vi "18_2.vi"() -> ()   [LabVIEW 2018]
panel:
  out "spreadsheet string":string="8\t*\t(\t3\t+\t6\t)\t*\t8\t*\t(\t2\t+\t4\t)\r\n"
  out "Value Out":u64=3456
  out "Operators 2":string[](array[string])=["8", "*", "(", "3", "+", "6", ")", "*", "8", "*", "(", "2", "+", "4", ")"]
  out "Array":u64[](array[numeric])=[86918496042, 35, 42033600, 5155488000, 1435, 231660, 320460800, 186, 2584012800, 1224608, 20280, 96, 28684, 4634, 288, 8798976, 155520, 2051315, 32682, 473128, 6966, 5107502736, 53084160, 1260, 204918052, 6900, 37044, 4092, 14580, 513010, 90, 123, 24752, 7920, 27216, 1360800, 28, 40960, 19296, 2934392832000, 33, 67469025, 9465, 114520, 5100, 637119, 654, 30, 2095120, 213355479168, 11827211, 6909, 26, 11328, 911680, 12644, 33, 207176, 4759, 1114344, 29, 12496275, 1118880, 520, 146480, 23520, 985600, 170311680, 156909312, 18, 180, 8456616, 50544, 75888, 6450672000, 1714006008, 12600, 36310, 24, 6604431, 982652496, 41920, 23328, 8400, 24524800, 32580, 1425, 2843, 27876736, 576, 114057, 17892, 18, 144720, 5882, 177600, 500, 4368, 190728, 303156, 39618, 75, 8640, 18, 1497233808, 112, 1188, 657720, 176904, 15750720, 3680, 832944, 1020096, 14696640, 29428, 918600, 23328, 4095, 125244, 19684, 7700400, 349930800, 2484, 3060, 9014208, 53844, 32480, 1190, 16224024, 5552064, 23997024, 176, 10032336, 41606712, 48, 159667200, 759974400, 318780, 2204, 87611717952, 608107500, 125, 126, 2880, 38, 8064, 30305, 500957184, 14675814, 19989504, 2278, 3030660, 212284816, 4105092, 536, 52995735016224, 7632, 18467906688, 9367068, 570381, 3933, 44335104, 546, 15120, 91887348, 34699, 2421, 252, 62008139, 240, 68094, 516, 123480, 81518400, 84, 85, 32702292, 560, 189, 115200, 83175, 49, 6480, 8603364, 3732, 282640, 48, 204880, 3594384, 340, 314230, 4608, 1890, 102920, 255143, 83520, 50, 124800, 47382618729600, 38, 311216400, 9856, 152611279793280, 3740, 24, 58432, 22804, 1168, 1200558240, 243000, 3123394014, 155, 1049280, 11383672, 18360, 4050, 1306384, 16698, 1392, 29664, 1400, 42912, 12096, 218601, 20352, 11520, 208, 290306, 10080, 51417, 32, 10320, 302702400, 35426, 380160, 1650, 1616630404200, 1725456, 6048, 12980, 34819572, 13600651680, 3616, 58, 21735, 294, 144, 59346, 590733000, 1636752, 138240, 56026441240, 1643, 1028160, 1430, 36000, 88185240, 530838400, 18304, 6921193, 5250, 8, 2002910, 240, 21345009840, 928, 12355200, 606060, 189800, 109188, 1312, 3512008281600, 6977998264320, 44528, 2898, 82560, 1271808, 55399939, 270, 139689930240, 918778, 31299840, 178560, 343245, 137511, 270, 62974800, 109192050, 9036, 5040, 15271200, 449592, 116701568, 38088, 1260, 269954916, 2388, 46824960, 6028, 173892, 12348, 24570, 20790, 814, 1834, 4651101, 272268, 799029, 58480, 68510, 3149120, 3224592, 303408, 368640, 29694467, 2690552148480, 30249, 1068480, 54966739968, 137280, 2640, 1071616, 70025904, 232190, 1470, 790, 2352, 3636, 4368, 53032320, 60984, 52564909320, 30151, 1751137542, 13272600, 10969, 48934553310720, 160524000, 4352, 31, 2450, 453648, 468, 257, 6426, 21560, 3466935, 648, 6552, 2536, 93148, 6538860, 41472000, 17988, 1366740, 816, 718502400, 228750, 13547520, 33564, 48681, 78624, 98385477120, 1826496, 26880, 321672, 23294304, 2205, 248371200, 8709606, 16496865, 276, 1451526, 18630, 14871, 152460, 14136304, 420, 945, 5265, 3456]
  out "sum":u64=320536571743074
  in  "Input":string="(7 * (7 * 6 * 4 + 3)) * 3 + ((8 + 5 * 3 + 7 + 8) + 3 * (2 + 9 * 5 + 7 * 5 * 6) * 2 + 3 * 9) + (4 + 5 + 5 * 2 + 2) + ((5 + 6 + 9 + 6) + 3 + 4 * 6 * 5)\n7 * 5\n(9 * (9 + 7) * 7 + (4 + 5 * 5 + 2 + 3) + 3) * 7 * 5 + 8 + (4 + (7 + 9 + 6 * 9) * 2)\n((6 + 4) * 6 * (5 + 3) * 9 * (3 * 5 * 5 * 9 * 4 + 9) * 4) * 2 * 8 + 9\n7 * 7 + (9 + 2 * 9 + 9)\n9 + (7 * 7 * 5 * 9 * 7) * 2 + 3 * 3\n5 * (5 * (8 * 4) * 7 + 8 + 7) * (5 * (4 * 3 * 5 + 2 * 5) + (6 * 6 * 7 * 2 + 2) + 4) + (5 + 4 * 7 + 5 * 9 + 9) * 2\n((7 + 3 + 8) + (2 + 6 * 4 * 5)) + 8\n8 * (6 * 7 + 3 * (8 * 5 * 2 * 4)) * (3 + (5 + 5 + 6) * (4 * 3 + 7 * 5 + 7) + (3 * 5 * 9 * 3)) + 8\n6 + 4 + 8 + 4 * ((3 + 5 * 8) + 7 * 7 * 8 * 7 * 2)\n3 * (9 + 4) * (9 + 2 + 6 + 5) + 4 * (7 * 2) + 6\n4 * 6 + (8 + 3) + 7\n2 + (8 * (5 + 6 * 5) + 9 * 7 + (7 * 7)) + 5 + 5\n(8 + (5 * 7 * 3 + 6) + 8) * 8 + 6\n8 * 6 * 6\n8 * 6 + (9 + 4 * 5 * 3) * 9 * (4 * 2 + 6 + 7 + 4 * 8)\n(5 * 9 * 8 * 9 * 6) * 8\n7 * 5 + ((2 * 7 * 5 + 2 + 6 + 3) * 9) * 5 + ((2 * 2 * 4 + 3) * 5)\n(2 + 3 * 4 * (2 + 4 * 9 + 8) * 8) + 6 + 8 + 7 * 2\n3 + 7 + (3 * 4 * (8 * 6 + 8 * 8 * 2 + 9)) * 4\n9 * 9 + 9 + (3 * 7 * 9 * 4)\n(7 * 7 + (2 * 5 * 8) * 4) * 9 + (9 + 4 * 8 * (9 + 3 * 5 * 4 * 7 * 4)) + 3 * 3\n7 + 6 + 3 * 8 * 4 * (9 * 4 * (5 + 7 * 2 * 8 + 7 * 8))\n(7 + 2) * 5 * 8 + 6 * 2\n9 + 4 + (5 + (7 * 7 * 9 + 5) + 6 * 5 + 2 * (4 * 7 * 7 + 8 * 5 * 5)) * 2 + 2\n8 + 2 * 2 * (2 + (2 + 7 + 7 * 7 * 3) + 7)\n3 + 4 * (3 + 3 * 3 + 4) * 9 * 6 + 8\n((4 + 4 + 6) + (5 * 5 + 4 * 9 * 5) + 5) + 2 * 2\n9 * 5 * 6 * 2 + 6 + (2 * 9 + (2 * 3 + 4))\n(3 * 9) + 2 * (2 * 5 + 7 + 9 * 7 * 6) + 5 * 5 * 2\n7 + 3 + 5 * 6\n7 + 5 + (2 * 8 + (6 * 6) + 6) + (4 + 7)\n2 * (9 + 5 * 3 + 5 + 5 + 4) * (3 + 4 + 3 + 5 + 2 + 7) + 2 * 2\n(4 * 5 + 6 * 3 + (5 * 3)) * 5 + 5\n9 + 8 + 7 * (7 + 9 + 2 * 2 + 7) * 7\n3 * 3 * ((4 + 3 * 4 * 2 * 2 * 6) * (9 + 6) * 3) * 5\n9 + 6 + 7 + 6\n8 * (4 * 8 * 8 * 7 + 4 + 9)\n2 + (7 * 9 * 2) + 6 * 6 * 4 * 6\n((4 * 6 + 7 + 9 * 4) + 9) * 4 * ((6 * 3 + 3 + 9 * 7) * 8 * 4 * 5 * (2 * 6 * 8 * 5 + 5 * 3)) * 7\n(4 * 7) + 5\n6 + 9 * 6 + 9 + ((5 + 7 * 5 * 8) + 7 + 7 + 8 * (2 + 8 * 2 * 4 * 7 + 9) * 7)\n6 + 3 + (9 + 6 * (4 + 7 + 4 * 6 * 7)) + 6\n5 * 7 * (4 * 6 * (3 + 8 + 6 * 8)) + 8\n(5 * 6) * 8 + 2 * 3 + (7 + 4 + 3)\n3 + 4 * 9 * 2 + (7 + (5 * 9 * 7 + 7 * 4) * 4) + 3\n2 * 9 + ((3 + 5 + 2 + 9 * 9 + 6) + 4 + (6 * 4) + 2) + 3\n3 + 6 + (3 + 6 + 8 + 2 + 2)\n8 * ((8 * 6) + (7 + 2 * 2 * 2 + 4 * 3) * (9 + 8 + 4 * 8) + 8 * 4) + 2\n9 + 4 * (7 * (2 * 4 + 9 * 3 + 7) * 8 + (4 * 3 * 9 + 9 * 5 + 7) + 9 * (6 * 4 * 2)) + ((5 + 6 + 7 * 9 * 6 + 6) + (6 * 2 + 8 + 9 + 4 + 4) + (8 * 5 * 2 + 6 + 7) * 5 + 3) * 9 * 8\n9 + 2 + (5 + 3 * 2 * (7 + 4 * 5 * 5 + 3 * 7) * 8 * (5 * 6))\n7 * (3 + 3 + 7 * 7 * 9) + (2 + 5 * 6 * 4)\n9 + 8 + 9\n8 * (7 + (5 * 7) + (7 + 3) * 2 + 7) + 4 * 3\n2 * (2 * 6 + 5 * 7) * 2 + (3 + 3) * ((2 * 3 + 2) + (5 * 3 * 4 + 8 * 2))\n4 * (3 + 7 + 6 + 8 + 3 + 6) + 8 + (2 * 3 * (5 * 2 + 6 + 5 * 8))\n2 + 5 + 3 + 2 + 4 + (2 + (6 + 4) + 5)\n2 * (4 * 4) + (5 + 2 * (4 + 2 * 2 + 4) * 4 + (5 * 9 * 9) + 2)\n(6 + 9 + (3 + 5 * 3) + 4 * 2 * 2) + 7 + ((6 * 6 + 4 * 5 * 5 + 4) + 5) + ((8 + 4 + 9 * 8 * 9 + 2) + (7 + 2 + 9) + 4) + 5\n7 * 3 + (6 + (8 * 5) * 6 * 8) * 2 * 9 * 4\n9 + 9 + 9 + 2\n(7 * 9 * 2 + 8 * 7 * 4) + 9 + (9 * 6 * 9 + 7) * 3 * (9 * 5 * 5)\n4 * 7 * ((7 + 9 * 5 * 4 + 7 * 4) + (2 + 3 + 5 * 4 + 2) + (2 + 5 * 8 * 5 * 5 + 6)) * 6\n5 + 8 * (9 + (9 + 3 + 9 + 5 + 5))\n(3 * 7 * 2 * 3 + (8 + 8 + 3 * 9)) + 8 + 8 * 6 + 8 + 6\n9 + 4 + 8 * (7 * 8 + 8 + 4 * 8)\n2 * 9 + 2 * (5 + 3) * 2 * (5 * 5 * 8 + (3 + 4 + 4 + 5) + 4 * 4)\n5 * 7 + 2 * ((2 * 8 * 8 + 8 * 2 * 7) * 6 * 7 + 7 + 2) * 2 + 9\n4 * (6 * (6 * 3 * 3)) * (7 * 5 * 4 * 2 * (5 + 5 + 8 * 3)) + 7 + 7 * 8\n3 * 2 + 4\n9 + 6 * 2 * 4 + 2\n((5 * 5 + 3 + 7 * 2) * 2 * 5 + (9 + 9)) + 3 + 6 * (9 + 8) * 8 * 9\n4 * (8 + 2 + 3 * 9 * 6) * 6 * 3\n2 * (9 * 6 + (8 + 6 * 4) * (5 * 5) + 9 * 2)\n6 + (3 * (6 * 6 + 4 + 5) + 3 * 5 * 4 + (6 + 9 + 4 * 5 * 3)) + 6 * (3 + (6 + 5 + 5 + 6) * 8 + 8 * 4) * 4 + 6\n9 * 9 * 2 + (6 * 4 * 2 + 4 * 7 * 9) * 7 + ((5 + 6 + 7 + 7) * (7 * 3 + 9) + 9)\n(2 + (6 + 8 + 6 * 5 + 5) + 8 * 5) * 9 + 3\n2 * 9 + 2 + (9 * (4 + 6 + 4 + 2) * 9 * 5 + 7 + 2)\n8 + 6 + 4 + 6\n3 + ((6 * 4 + 2 + 4 + 3 + 8) * (4 * 3) * (9 + 4 * 6 + 2 * 7 * 6)) + 5 + 7\n3 * (8 * 4 + 9 + 4) * 7 * 2 + ((5 + 9 * 6 * 4 * 4) * 8 * 4 * (6 + 2))\n((8 * 7 + 6) * 3 + 2 + 5) + 8 * 5 * 8\n(3 * 2 * 6 * 3 * 2) * 6 * 2 * 9\n(4 * 8 * 3 + 5) + (8 + 9) + 7 * 7 + 3 * 3\n(2 + 7 * (7 * 8)) + 8 + (6 * (4 * 8) * 4 * 2 * 8) * 4 * ((7 + 8 + 4 + 3 + 6) * 4 + 9 + 4) + 3\n((7 + 2 + 3 * 3) * 5 * 5 + 4) + 9 * 2 + 7 + 9 + 2\n(6 + (2 + 7)) * 4 + 7 + 8 * 5\n(9 * 8) + (8 + (2 + 4 + 5 + 6 * 9) + 2 * (8 + 9))\n2 * (9 + 8) * 8 * ((7 * 6 + 7 * 3) + 2 + 5 * (7 * 2 + 7 + 8) + 3 * 3) + 8\n4 * 6 + 6 + 4 * 9\n(2 + 4 + 5 + 3 + 6) + 3 * 3 * 3 + (5 * 2 * 9 + 6 * 6 + 5)\n7 * 5 + (6 + 2 * 2 * 8 + 5) * 6 + 6\n(5 + 8 + 2) + 3\n3 + 3 * 5 * ((3 + 8 + 5 + 9) * 4 + 4 * 4 + 4) + 8 * 3\n2 + (5 + 5 + (6 * 5 * 2 * 8) * 4 + 8)\n8 + (5 * 7 * 2 * 2) * (7 + 9 * 5) * 2 + 9 + 4\n((9 * 9) + 6 + 4 + 9) * 5\n5 + 3 * ((4 + 8) + 9 * 2 * 6 + 7)\n6 + 7 + 5 * (2 + 9 * 4 * 5 * 7 + 5) + 9 * 4\n(7 * 2 + 4 + (8 * 8 + 2 * 5 * 3 * 6)) + (4 + 4 * 3 + 7) + 4 * 6\n2 * (5 * 9 * (5 + 3 * 5) * 5 + 6) + 4 + 5\n5 * (4 + 7 + 4)\n9 * 7 + 8 + 4 + (6 * (6 * 2 * 4 + 9)) + 5\n6 * 3\n(5 * 6 + 2 * (2 + 5 * 6 * 4 + 9 + 2)) + (4 + 3 * (9 * 9 + 4 * 8 * 8 * 9) * 4) * (8 + 7 + (4 + 8 * 2 + 4) * 9)\n8 * 5 + 9\n7 + 4 * 9 * 6 + 6\n9 + 6 * (8 * (7 * 6 + 2 + 4 + 6 + 9) * 2 + 2 + 2 + (7 + 7 + 9))\n6 * (7 * 6 * 6) * 9 * 6 + 7\n(5 * 7 + 9) * 7 + ((4 * 5 + 3) * 5 * (3 + 8 * 7) + 2 + 3 * (7 + 6 + 2)) + (3 * 5 * 5) + 2\n4 * 2 * 2 * 2 * (6 + 4 + 9 + 4 * 5)\n((9 * 7 + 7) + 8 * 7) * 4 + (7 + 9 * 9) * 6\n8 * (6 * (8 + 4) + (5 + 6) * 6) * 7 + 4 * 7 * 2\n(7 + 7 * (8 * 5 + 4)) * 5 * (3 * 6 * 2 * 3 * 9) * 3\n4 + (7 * 5 * 3 * 5 + 3 * 5) * 7\n(6 + 5 + 6 * 3 * (6 * 4 + 6)) + 2 * 5 * 9 + 3 * 5\n3 * (6 + 3 + 5 * 3) + 6 * 3 + (7 + 8) * 9\n(3 + 8 + (5 * 4 + 4 + 7) + 5 * 2) + 2 + 5 + 6 * 9 + (4 + 2 + 6)\n9 * 8 + (3 + (4 + 2 * 8 + 7 * 5 + 3) + (3 * 3) * 3 + (2 * 8))\n7 * 4 + (3 + 7 + 6 + 4 * (3 * 6) * 2) + ((5 + 5 * 5) + 6 + 2 * (2 * 3 * 3 + 3))\n9 * 5 * (6 + (2 * 3)) + (3 * 4 + 3 + 9 + 6) + (9 + 5 + 2 + (3 * 4 * 9 * 9 * 5) + 2 * 7) * 5\n(6 + 9 * 4 + 5 * 4 * (8 + 2 * 4 * 2 * 3)) + 4 * 9 + 6 * (4 * 5 * 9)\n9 * 7 + (2 + (6 + 3) + (4 * 3 + 9) + 9) + 8 + 9 * 3\n3 * (8 + 7 + 7 + 8) * (5 + 5 + 2 + 6 + 9 + 7)\n7 + (7 * 5 + 3 * 4 * 9 + 2) * (8 * 6 + (5 + 2) + 6) * 4 + (6 * 3) + 2\n(4 * 5 + 7 + 3 * (7 * 8) + 8) + 6 * 2 + 9 + 3\n7 * 4 * 8 * (7 + 5 + 2) + (8 * 8 * 2) + 3\n7 + 7 * (6 + (4 * 7 + 3 + 2 + 7) + 3)\n2 + (8 + (5 + 9 + 2 * 6 * 6 + 8) * 8 + 2 * (5 * 2 + 8) * 4) + 2 * 6\n(4 * 9 * (7 * 6 * 9 + 8 * 6) * 9) * 2 * 2\n3 + (8 + 2 + (2 + 3 * 2) * 6 + (5 * 8 * 8 * 8 + 2 + 3)) * 4 * (9 + 3) * 6\n8 + 3 * (3 + 5) + 3 + 5\n4 + ((9 * 5 * 2 + 7 + 5) + 6 + 3 + 6 * (7 * 6) + 6) * 2 * 3 * (3 * 9 + 9)\n((4 * 9) * 8 * 6) + 8 * 8 + 6 + ((6 + 4 + 7) * (2 + 2 * 4 * 9) + 3 + (5 * 9 + 9 * 9 + 5) + 2)\n(8 * 4) + (8 + 8)\n((4 + 5 + 2 * 4 * 7 + 3) * 6 * (4 * 6 + 8) * 9 * (9 + 7 + 5 + 3)) * 5\n8 * 2 + 8 + (7 * (8 + 2 + 6 * 7 + 9) + (5 + 9 + 3) + 6 * 6) * (8 + (4 * 2 + 4 + 7 * 5) + 2 * 6) * 5\n(2 * 5 + (8 * 7 + 9 + 2 + 2)) * 2 + (8 * (2 + 4) + 4 * 5 + 7) + 4\n4 + (2 + (4 * 3 * 9) * 5 * 4)\n((3 + 4) * 7 + 6 + (5 * 3 * 8 + 8 * 9) * 3 + 6) + 8 * 4 * ((7 + 4 * 3) * (6 + 9 + 9 * 4 * 7) + 9 + 5 + 2 + (5 + 8 * 4 * 6 + 4 * 8))\n4 * (9 * 5 * (5 * 7 * 7 + 4)) * 5 * (5 * 7 + (4 * 5) * 4 + 9)\n5 + (8 * 6 + 8) + 8\n7 + (8 + 6) * 4 + 2\n(3 * (9 + 6 * 8)) * 8\n3 + 6 + 4 + ((5 + 4 * 2) + 7)\n7 * 3 + 5 * (2 * 5 + 4) * 8\n5 * 5 + (6 * (8 + 5) * 7) * 7 + 4\n7 + 9 + (2 + (3 + 8 + 4) + 9 * 2 + 6) * (7 + (3 + 6 * 8 + 8 * 7) + 9 * 3 * 8 + (9 * 6 + 2 + 8 + 4 * 4))\n6 * (2 * 8 + 3 + 5 + 5) + (3 + (8 * 2 * 3) * (2 + 9 * 8 * 5 + 3) + 4 + 7) * 7 + (5 * 5 + 7)\n(2 * 2 * 6 * 4 * 9 + (9 * 5 + 7 * 4 + 6 * 2)) * 4 + (4 + (8 * 2 + 3 + 6))\n2 + (8 + 4 * 8 + 3) * 6 + 7 + 4\n(6 + 6 * (2 * 5 * 5 * 4 * 5 * 4) + 8 * 7 * 3) + 5 + (3 * 6 + 3 * 7) + 5 + 5 * 3\n2 * (8 + 2 + 6 * (9 * 9 * 9 + 4 * 2 * 7) * 3 * (4 + 6 * 3 + 8 + 4)) + 8\n(6 * 7 + 8 * 6 * 7 + (5 + 9 * 3 + 6 + 9 * 5)) + 2 * 6\n(7 + 2 * 4 + 3) + 4 * 5 + 3\n((7 * 7 + 2 + 7) + (3 + 3 + 5 + 9 * 3 + 2) * (2 * 4 * 7 + 6 * 3)) * (2 + (7 + 4 + 3 * 9 + 4 * 5) * 4 + 3 * (5 + 8 * 3)) + 5 + (2 + 8 * 2 * 8 * (6 * 7 + 4 + 5)) * (3 * (7 * 6 * 3 * 8)) + 7\n3 * 4 * ((8 + 8 + 9) * 6 + 6 + 7 + 6) + 8 + 3\n(6 + (7 * 4) + (9 + 6 + 3 * 9)) + 2 * (4 + 6 * 5 + (2 + 8) * 5 + 9) + 3 * (6 + 8 + 8 * (7 * 8 * 3 * 2 + 2 + 8))\n(9 + 8 * 4 + (5 * 8 + 7 * 2 * 8 * 9) * 8 + 9) * 3\n9 + ((5 * 3 + 6) + (8 + 6 * 6 + 7 + 2 + 8) * 8 + 5 + (9 + 8 + 2 * 9 + 2)) * 7\n((8 + 2 + 6 + 3) * 8 + 5 + 8 + 2) * 9\n(6 + (4 * 4 * 7 * 2 + 6) * 4 + 2 * 8 * (6 + 2 * 8)) * 2 * 8\n3 * (4 + 3 + 3 + (3 * 7 * 7)) + 6 + 7 + 4 + 8\n(6 * 8 + 7) * 8 * 9 + 8 + 4\n(7 * 7) * 2 + (8 * 7) + 4 * (5 * 2 * (3 + 4 + 7 * 8 * 3) * 9) + 6\n7 + (9 * (6 + 8 * 7 + 6 * 3) + 4) * 4 + 3\n6 + 3 * ((2 + 2 + 3 + 9 + 9 + 8) * 6 + 2) + 5\n3 * 6 * 6 + 2 + 2 + (2 * 2)\n6 + (4 + 9 * (5 + 9 * 4 * 6 + 6) + 4 * 6 * (2 * 7 * 7 * 4 + 8)) + 5\n((2 + 6) + 2 + 5) + 7 + 3 + 5 * 3 + 5\n(6 * (2 + 8 + 7) + 4 * (2 + 8) * 9) + 9 * 6\n(2 * (9 * 4 * 3 * 2) + (4 + 4 * 3 + 2)) + 4\n(6 + 4 * (5 + 9)) + 7 * 7 * 8 * 5 * 3\n(3 + (5 + 4 * 3 + 9)) * 2 * (9 + 6 * 6 * (7 + 8 + 2 * 5) * 8 * 6)\n8 + 6 * 6\n8 + (8 * 9) + 5\n8 + (7 * (6 + 8) * 7 * (5 * 7 * 8 * 7) + (8 + 4 + 6 * 9 + 8) + 4) + (6 * 4) * 3 * 7\n9 + 4 + 3 * 7 * 5\n(8 + 9) + 6 + 4 * 7\n5 * (4 * 6 + 4 + 2 * (5 * 2 * 2 * 8)) * 3\n3 * 3 + 2 + ((8 + 5 + 4 + 8 + 8) * 7 * 6 + 9 * 8)\n9 + (8 + (8 + 9) + 7 + 8)\n(8 + 2) + (2 + 5 + 7) + 6 * 6 * 6 * 6\n5 + 7 + (5 + 4 * (5 * 6 + 3 + 3) + (7 * 9 * 5 * 6 * 6 + 3) * 8) * 7\n6 + ((7 * 3) * 6 * 5 + 5 + (3 + 3 + 9)) + (6 * 2 + 6 + 9 + (2 + 4 * 3 * 4) + 7)\n8 * 5 + (9 * 2 * 7 * 2 * 6 + 8) * 2 + 2 + 6\n6 * 8\n(2 * 3 + 5 + (8 + 6 * 8 * 7 * 2)) * 3 + 2 + 6 + 2 * 5\n(7 + 6 * (2 + 2 * 4 * 9 + 7 * 5) * 4 + 2) + 4 * (9 + 6) + (9 + 5) + 7\n5 * (3 + 7 + 7 * 4)\n2 * ((2 * 7 * 8 * 4 * 3 + 7) + 6 + 3) * 5 * 7\n8 * 4 + 7 + (6 * 4 + 3 + 2) + 7 * 8\n7 * 9 + (2 * 9 * 2) * 6\n8 + (6 * (2 + 8) + 9) + (7 + 6 + 6 * (8 * 3 * 5 * 5 * 9) + 3 + 7) + 8\n2 + 5 * 4 + (4 * (3 + 7 * 5 + 8) * 8 + 2) + 3 * 7\n(8 * (9 * 7 + 9 + 9 + 4) * 3 + 2) * 8\n4 + (6 + (2 + 4 * 6) + 4)\n(8 * (4 + 6 + 2 * 6 + 7)) * 9 + 8 + 3 * 5\n((2 * 7 + 3 * 5) * (5 + 7 + 7 + 3 * 7 * 3) * 8) * 2 * ((2 * 9 * 4 * 6 + 4) + 6 + (8 * 5 * 4 * 5 * 6 * 8) + 7 * (9 * 6 + 7 * 3 + 4 + 7)) + 9\n6 + 8 + (3 * 3 + 2) + 5 + 4\n5 * 6 + 6 * 5 * ((3 + 5 * 8 + 4 * 8) * 9 * 9 + 6 * 4 + 6) + (4 * 7 * 5 + 9 + 7)\n2 * 7 * (4 * 7 + (4 + 7 + 4 + 3 * 2 + 7) + 7)\n((8 + 3 * 6 * 6 + 4) + (9 + 5 + 3 * 3) + 7 * (3 * 4 + 4 + 9 * 4 + 6) + (8 + 5 + 2 * 2 * 5)) * 8 * 6 * 7 + ((5 + 6 + 2 * 4 + 2) * (9 + 8 + 9) + 6 + (6 * 5 * 9 + 7) * 4 * 6) * 7\n4 * 5 * (9 * 3) + (9 + 6 + 5 * 8)\n3 * 8\n9 + 2 * (7 + (2 + 9) * 9) + 4 * 4 * 8\n(8 + 4 + 7 * 2 + 8 * (8 + 7 * 4 + 4)) + 4\n4 + 8 + ((7 * 9 + 9) + 3 + 2 + 3) * 8\n(6 + (4 + 3 + 8 + 6 * 8)) * (5 + 9 * (5 + 2 * 7 + 8) + (6 * 7 * 4 + 2 * 5) + 4 * 9) * 8 * 5\n8 + 3 + 4 * 9 * ((4 * 9 + 3 + 6) + 3 * 3 + 9) * 2\n6 + ((3 * 2) * (4 + 9 + 9 * 5 * 2) * (2 * 8 + 4 * 7 + 4 + 8)) * 5 + (9 * 4 * 6 + 6 * 4 + 8)\n2 + (5 + 4 * 8) + (9 * 9)\n8 * 3 + 7 * 3 + ((2 * 2 + 6 * 3) * 3 * 7 * 8 + 5) + 9\n4 * 7 + ((6 + 7 * 3 * 4 + 8) * 2 + 6 + (4 * 6 + 9 + 6 * 8 * 3) + 3 * 3) + 3\n5 * (9 * 9 + (7 + 6 + 2 + 9 + 9 + 9)) * 8\n5 + 4 * 2 + 7 * (5 * 5 + 2 + 3)\n2 * 2 + 6 + ((2 + 2 + 5) * 6 * (2 + 7 + 3 * 9) * 5 + 9 * 8)\n((2 * 4 + 7) + 9 * 8) + 5 * 6 * 2 + 9\n6 + ((7 * 9 * 9 + 2) * 2)\n6 * (7 + (4 + 7 * 2) * 5 + 2 + 7) + 6 * 7 + 5\n8 * (6 * 8 + (7 + 2 + 7) + 3) + 7 + 6\n(7 * 2 * 3 * 7) + 4 * 3 + 6 * 9 + 7\n8 * 7 * (8 * 9 * 3)\n9 + (9 * 4 * (9 + 3 * 5 + 9 + 9) * 8 + 5 + 9)\n6 * (9 * 2 * 9 + 6 + 9 + 8) + (6 * 9 * 5) + 2 * 4\n2 * 5 * (7 + 8 + 3 + 8 + 6 * 4) * 4 + 5\n2 * 2 * (4 + 3) + 2 + 4 * 4\n(6 * (9 * 6 + 2 * 2) * 4 * 3 * 4 * 7) + 2\n(2 * 5) * 3 + 3 * 3 * 7 * 8\n3 + 6 + ((6 * 6) * (9 + 8 * 2) * 7 + 5 + 9 * 2)\n9 + 7 + (2 * 8)\n(8 * 7) + (8 + 6 * 7 + (3 * 9 + 6) * 6 + 8) + (4 * 2 * 9)\n2 + 2 + 2 + 9 * ((4 + 5 * 7 * 5 * 4 * 7) * (9 + 9) + 4 * 4 + 9) * 8\n4 + 2 + ((6 + 8 * 4 + 7) * 7 + 3 * 9 + (9 + 5))\n7 + 8 * (3 * (3 + 9 + 6 * 5) + 6 * 8) * 7 + 4\n8 + 7 * (2 * (5 * 7)) + (4 * 3 + 7)\n(2 + 8 * 7) + ((8 * 9 * 3 + 3 + 5 * 7) * 2 * (9 + 6 * 3 * 5) * 4 * (4 + 6 * 6 + 4 * 9) * 3) * 6 + 4 * 4 + 2\n3 * (9 + 4 + (9 + 5 + 8 + 6 * 3 * 4) * 8 + (9 * 3 + 8 + 4 + 7)) * 8\n(4 + 4 * (4 * 7)) * 2 + 7 * 3\n((4 * 9) * (9 + 6 + 9 * 8 + 7)) + 6 + 7 + 7\n6 + ((9 * 5 + 9 + 6 * 6 + 4) * 7 + (9 + 5 + 5) * 9 + 3) * (5 * 9) + 8 + 9\n(3 + 8 * (7 * 3 * 4)) * (6 * (6 + 4) + (9 + 8) * (2 * 5 + 4) + (8 + 5 * 6 + 5 * 2 + 2)) * 6 + 9 + (7 + 6 * 5) + (5 + 4 + (6 + 8 * 2) * 2)\n4 * ((6 * 8 + 7 * 6 + 4) + 4)\n((5 * 6) + 4) + (9 + 4 + 9) + 2\n5 * 9 * 7 * 6 + (9 * 7)\n5 + (2 + 7) * 5 + 9 + 7\n6 * 2 * 8 + 4\n(3 + 2 * 4 + 8) + ((7 * 5 + 7 * 2 * 8) + 7 + 2) * 6 * 2 + 5\n(2 * 5) * (3 * 9 * 4 * 8 + 5 * 3) * ((9 + 5 * 6 * 3) + 3 * 7 + 4) * 5\n((3 + 6 * 3) * (4 + 9 * 5 * 6 + 4 * 7)) + ((8 * 7 * 2 + 7) + 5 * 6) * 6 + 7\n(8 + 4 * 8 * 8) * 9 * 9 + 7 + 4\n(7 * 9 + 5) * 5 + (9 + 4 + 4 + (7 * 9 * 2 * 8 * 2 + 9)) * ((7 * 5 * 7 * 3 * 7) * 5 * 2) + 8\n5 + (6 * (8 + 9) * 7 + 9) + 3 + 3\n8 + 8 * (6 * 5 * (3 + 5 + 9 * 2 * 9 * 7))\n5 * (4 + 7) * 5 + 7 + 8 + 6\n3 * ((5 + 6 + 2 + 7) * 4 * 6) * 5 * 5\n(6 + 3 * (9 * 9 * 7 * 8 * 9 + 9) + 5) * 8 * 6 + 7 + 2\n8 * (4 + 3 * 5 + (5 + 2 * 3 + 8) * 2 + (8 + 7 * 7 + 4 * 7 + 7)) + 8 * 6 + 4 * 5\n4 + 7 * 8 * (2 + 6 + 5) * (4 + 8 + 4)\n9 + 8 * ((2 * 3 * 6 + 4 * 2) + (6 * 5 * 9 + 7) * 5 * 2 * 9 * 7) + (9 + 4 * (2 * 8 * 7) * 3 + (9 + 8)) + 3 + 6\n7 * 3 * 8 + ((6 + 7) * 9) * 2\n5 + 3\n4 + 9 * 7 * ((7 * 8 + 7 * 2 + 5 * 7) + 5 * 4) + (5 * 5 + (7 * 6) * 6)\n((2 + 4) * 5) * 3 + 5\n5 + (2 + 8 * 9 * 6 * 2 * (2 + 8 + 3 + 5)) * 9 * 8 + 3 * (9 + (4 + 2 + 4 + 7 * 4) * 9 * 9 + 7)\n2 + 6 * 9 + 3 + (7 + 8 + 2) * 4\n5 * 4 * (2 * 4 + 3 + 3 * (9 + 6 + 6) + (3 * 8 * 4)) * 4 * 3 + (9 * 7)\n7 * (5 * 5 + 4 + 8 + (3 * 4 + 6 + 9)) * 2 * 9 * (6 + 7)\n2 + (5 + 3 * 5 * 8) + 3 * 8 + (9 + 9 * 8 * 2 * 2)\n((7 + 9 * 9) * 7 * 2) + 6 * 6 * 9\n(6 * (9 + 9 + 4 + 5 + 6 + 2) + 6 + 8 + (7 * 3 * 8)) + 2 + 6 + 2\n(3 + (6 * 2 + 2 + 6 * 7 + 8) * 9 * 2) * ((2 + 9) + 8 * 9 + 2) + 3 * (3 + 4 * 7 * (3 + 2 * 8 * 6 + 7) * (5 + 3)) * 5\n(9 * (9 * 9 + 7 * 4) + (7 * 4 * 7 * 5) * (9 * 2 + 8 + 5 * 6)) * (6 * (7 + 9 + 6 * 7 + 9) + 4 * 4 * 2 + 6) * 9\n4 + (3 + (4 + 5)) + 7 * (6 + 4 * (5 + 3 + 9 + 5 + 2) * 4 + 4) + 8 + 8\n((5 + 8) + 5) * 9 + 6 + 8 * 7\n8 * (5 + (3 * 3 + 6 * 3)) * 5 + 2 + 8 * 8\n6 * 2 * 9 * (8 * 7 * (2 * 4 + 6 + 7 + 4 * 5)) + 9 + 7\n(5 * 3 * (8 * 2 * 8 + 2 + 8) * (8 + 8 + 9 * 7 * 6 * 3) + (4 * 2 * 7) * 4) + (4 * 3 + 9 * 5) + 5 + (5 + 9)\n(6 + 3) * 5 + (6 + 7 + 5 + 7)\n(9 * (6 + 6 * 8 + 4) * (3 * 6 + 6 + 7 + 7 + 5) + (5 * 7 + 4) * 9) * (7 + 3 + 7 * 2 + (5 + 7 * 6 + 8) * 4) * 7\n6 + 8 * (5 * 5 + (3 * 2 * 2 * 7 + 4 * 9) * 7 + 4) + 8 + 4\n9 + (5 * 7) * (5 * 6 * 8 * (5 * 2) + 9) * (6 + 3 + 6 + 9 + 2) * 6\n8 * (8 + 8 + 9 + 9 * 6 * 3) + 8 * (3 * 3) + 3 * 3\n7 * 7 * (5 + 5 * 9) + (6 * 6 * 3 * 4 * 8 + 8) + 3\n(3 * 2) + 5 * (6 * (9 + 2 + 3 + 2 * 9 + 5) + 6) + 2 + 7 * 9\n9 * 2 + 3 + (3 * 7) + 4\n7 * 5 * 7 * (4 + 3 * 7 + 3 + (4 * 5 + 5) + (5 * 8)) * (8 * 3 * (8 + 9))\n((3 * 8 * 8 + 6 + 5 * 5) + 3 + (3 * 8 * 7)) * 2 * (9 + (9 * 8) * 5) * 5 * 4 + 7\n4 * 9 * (4 + (3 * 7) + (6 * 4 * 9)) + 2 + 8\n5 * ((7 + 2 + 6 + 6) * 2 + 4 * 8)\n5 + 9 * ((7 + 2) * 5 * 4 * (5 + 7) + (8 + 4 * 8 * 7 * 9))\n((4 + 3) + 6 * 3) * (4 * (4 * 6) * 3 * 2 + 8 * 4) + 8\n5 + (6 + 3 + 6 * 8 * 7 * 2) + 3 * 9 + (8 + 2 + 6 * (4 + 6 * 6 * 8 * 3 * 3)) + 7\n7 + (8 + 8 * (8 + 3 * 3 * 5 + 2)) + 4 + (2 + 3 * 7 * 7 + 6 + 2) * 9\n7 * 3 * 2 + 6 + 7 * 4\n(3 + 4 * 7 + (8 * 3 * 5 * 8 + 5 * 3) * (7 + 4 * 8 + 9)) + 8 + (4 * 3 * 4) * (6 + 4 + 8) + 5 + (9 + 6 + 2 + 4)\n((3 + 9 + 5) * 7 * 2 * (3 + 7)) + 5 + 3\n(4 * 9 + 3 + 9) * 8 * 8 + ((7 * 2 + 6 * 2 * 2) + 8 * 3 * 2 + 2 + 6) * 3 + 7\n(5 * 6 * (8 + 8) + 2) + 6 + 2 * (5 + 4) + 2\n(3 * 8 + 2 + 5 + 6 + 6) + (8 + 7 + 9 * 4 * 4 + (4 * 4 + 4 * 7 + 7)) * 4\n(7 * 7 * 4) * 7 * 3 + 6\n(9 * 3 + 7) * 7 + 4 + 2 * 7 * 3\n6 * 9 + (6 * 6 + 6 * (3 * 9 + 7))\n5 + 6 * 7 + 8 + (3 * 3 + 5 + 3 + 6) + 8\n(6 + 4 + 6 * 9) + (3 * (6 * 3 * 2 + 2 + 9)) + (2 + 9 + 8 * 3 * 8 + 9) + 4 + (4 + 4 + 7)\n4 + 3 * ((6 * 3 * 2) + 3 * 3 + (6 * 4 + 5 * 5 * 7) * 6 + 3)\n2 + (7 * 5 * 6 + 8 + 4 * 8) * 3 * 6 * 3\n9 * (8 * (6 * 7 + 7) * 3 + 9) + 7 * 5 + 6\n((3 * 5) + 2 * 4 * 2) * 7 + (4 + (4 * 2 * 6) + 2) + (3 + 5 * 8 + 6) + (5 + 2 * 6) * 2\n8 + 9 * (4 + 6 + 9 + 2 + 4 + 6) * (9 + 4 * 5) * 2\n(6 + 9 + 4 + 7 * 7 + (6 + 5 + 4 * 6 + 4 * 5)) * 3 + 7 + (2 + 9 + 7 + 8 + 4 * 5)\n(6 * 7 * (7 * 7 + 3 * 9 + 4 * 2) + 8 * 7) * 3 * 2\n(7 * (5 * 2 + 2 + 8 * 4 + 6)) + 7 + 7 * 8 * 7 + 2\n(8 * 6 * (4 + 6 * 8 * 8)) * 8 + 4\n(4 + 7) * (7 * 4 + 4 + 5 + (9 * 9 * 4 * 5) + 8) + 4 + (8 * 9 + 2 + 4 * (2 * 2 + 8) * (5 * 7 * 4 * 6 + 2)) + 6\n4 * (8 * (2 * 5) + 4 * (7 * 2 + 7 + 8) * 7) * 4 * 9 * 7 + ((5 * 4 * 5 + 7 + 9) + 7 * 7 + (6 * 3 + 8 + 7 * 4) + (6 + 4 * 3))\n((3 + 4 + 7 * 8 * 5) * 9 * 6) + 6 + 3\n((7 + 3 * 8) * (3 * 7 + 4 * 3) + 5 + 2 * 9) * 8 + 4 + 2\n((3 + 8 * 8 + 9) * 5 * (5 * 6 + 5 + 7)) + 2 * (6 * 5 + 4 * 6 * 4 * 8) * 9 * 7\n4 + 9 * 8 * ((8 * 6) + 7 * 2 + 2 * 6)\n(2 * 3 * 3) + 4 * 8 * (3 * 5)\n(8 * (5 + 9) + (5 * 6 * 7 * 2) + 4 + 4 + (6 * 9 + 8 + 7 + 2)) * 7 * 2 * 6 + 2 * 2\n(8 * 9 * 7 + 3 * 6) + 5 + 4 * ((9 + 8) + (3 + 7 + 6 * 2) + (7 * 5 * 9 + 5) * 8 * 3) + (6 + 9 * (6 * 8) + 2 + 4 * 4)\n6 + 8 * 9 + (4 * (9 + 2 + 3 + 5 + 3 + 8) + (3 + 7 * 4) + 4 * 7 * (6 + 2))\n2 + 4 * 7 * 5 + (8 * 3) + 6\n9 + 9 + 4 + (4 * 3 + 3 * 2 + (7 + 2 + 9 + 8) + 4)\n3 * 7 * 7 * 9 + 7\n(3 * 2 * 3 * 5 + 6) + 4 * 5 + 8 + 5\n7 * 6 + 7 * 8 + 8 * 3\n(6 + 2 + (6 * 8 * 5) * 6 + 3 * (8 * 5 * 9 * 2 * 7 + 4)) * 3\n(8 + (4 + 2 * 3 + 7 * 5) * 9) * 3 + 9 + 4 + 6\n(9 + 6 + (6 + 3 * 2 + 8 * 5 + 7) + (8 + 8 * 3 + 9 * 4 * 8) + 6 * 2) * (7 + 9 + 5 + 8) * 7 + 4 * ((6 * 5 * 7 + 7 * 9 * 3) + (2 * 4 + 4 * 2))\n(5 * (3 + 5 + 5 * 6) * 7) + 8 + 3 * 4 + 7\n3 * 7 * (9 * 5 + 9 + 7) + 9 * (3 * 4 * 4 * (8 * 4 + 2 + 5)) + (9 * (5 * 3 * 4 * 9) + 5 * 8 + 9 * 5)\n6 + 7 + ((2 * 4 * 5 + 7) * 2 * (8 + 8 * 4 * 3) * 3) * 5 * 6 * 4\n7 * (9 * 6 * 4) + 7 + (8 * 2 * 7 * 4 + 8)\n4 + 7 * (8 * 4 * 2 * (2 + 5 + 9 + 5 * 2 + 5) * (5 * 6 + 2 * 5 + 9) + 3) * 9 * (3 * 6 + 3 * (4 * 4 * 6 + 6 * 2 * 9)) + 8\n2 + 6 * (8 + 9 + 6 + 2 * (9 + 4 * 7 * 5 + 5)) * (7 * 7 * 2 * 9)\n4 * 3 + (8 * (6 * 8 + 8 + 6) + 3) + 5\n(5 + 6) + (2 + 6 + 4 + 8)\n(9 * 5 * 3 + 6 * 6) + (5 * 4)\n3 * 2 + (7 + 7 * 2 + (6 + 6 + 2 * 8 * 4) * 3) * 8\n(4 * 6 + 6) + 4 * 9\n6 + (9 * 3 * 3 * 3) + 8\n(5 + (9 + 6 + 3 + 7 * 3 + 5)) + 5 + (4 * 3 + 4) * 9 * 3\n(6 + 8 * (8 + 3 * 2 + 4 + 5 + 9)) * 7\n6 + 3 * 3 * 5 + ((7 + 4 * 8) + 2 * 7 + 4 * (5 + 8) * 8) + ((5 * 4 * 2) * 4 * 5 + (3 + 4 + 4 * 7 + 7))\n2 * 3 * 3 * 4 * 7 + 2\n6 * (7 + 9 * 9 + (9 * 6) + 5) + 4\n8 * (2 * 7 + 5 * 5 + 8) + 5\n(4 * 5) + (3 + 3 * (5 * 9 + 8 * 2) + 6 * 4 + 4) * 5 + 6\n4 * 9 + (3 + 3 * 2 + (2 + 4 * 4 * 7 * 7 + 5) * 9) * 5 * 3\n(5 * 3 * 6 + 8 + 2 + 4) * 6 * 8 * ((6 * 2 + 2 * 4 + 6 * 2) * 6)\n4 * (5 * 4 * 6 + (7 + 3 * 9 + 3)) + (3 * 4 + 4 + (5 + 7 * 6 * 2 + 7) + 3)\n3 * (5 + 2 * 6 + 8 + 5) + ((8 + 3 * 6 + 8 * 3) * (7 * 7)) + 8 * 4 * 5\n4 + (8 + 6 * (4 + 3)) * 4 + 4\n4 * 3 * (3 + (8 * 9) * (9 * 7 * 4 * 9 * 4 * 8) * (5 + 2 + 2 + 2))\n8 + (2 + 2 * 5 * 3 * (4 * 3 + 7 + 6 + 3)) + 7 * 2 * 5 * 5\n4 * (7 * 9 * (2 * 2 * 5) + 2 + 8 * (6 + 2)) * 4 * 7 * 8\n(2 * 3 * 3 * 2 + (9 * 8 + 5 + 4)) + 7 * 2 * 6\n((6 * 7 + 3 + 3 * 4) * (5 + 9 + 5) + 7 * 6) + 9\n6 * 9 + 8 + 3 + 6 * (6 * 9 + 9 + 3 * 2 * 2)\n(3 * 5 + 2 + 9) * (6 + 9 + (6 * 8 + 2 + 8 * 3 + 8) + (2 + 6 + 6 + 6 * 3)) * ((7 * 5 * 9) * 3 + 9 + 3 + 8 * 2) * 8 * 6 + 8\n3 * (4 + 4 + 6 * (5 + 7) * 8) * (3 * (6 * 7 + 3 + 7 + 7) + 7)\n6 * 8 + 8 * (6 + 9 + 5) * 7 + 7\n3 * (8 + 5 + 8 * 7 * 7 * 8) + 7 + 9 * 4 + 9\n(4 + 5 + 7 + 6) * (9 * (6 * 3 + 9 + 3 + 3) + 6 * 8 + (2 * 8 * 4 + 7 + 5 * 4))\n7 * 2 + 3 * (5 + 9) + 7 * 3\n7 * 8 + 5 + 7 * 4 * ((7 * 4 + 8 * 8) * (6 + 5 * 8 + 7 + 5 * 3))\n(7 * 4 + 3) + (7 + 9 * 7 * 9 * (3 + 2 * 2 * 8 * 2 * 6)) + 5 * 3 + 3 + 3\n5 + 6 * (3 + 6) * (6 + (7 + 2) * 3 + (8 * 6 + 3 + 8 + 5 * 9)) * 7\n(9 + 6 + 8) + 3 + 5 + 2 + (3 * 9 + (8 + 3) + 7 * 3)\n6 + (9 + 7 * 2 * (8 * 9 * 2 + 7 + 6 * 7) * 6)\n2 + 4 * ((7 * 2 + 4) * 8) + 9 * 3 * 3\n3 + ((5 + 4) * 4 * 7 * (3 + 5 * 4 + 3) + 3)\n(7 + 4 * 3 * 6 * 7 * 5) * 2 * 7 + 4\n(7 * (7 * 9) + 8 + 2 * (6 + 9 + 9 * 2 * 5) + 7) * 7 * 7 + 9\n(2 * 5 + 9 * 5) * 3\n3 * 9 + 5 + 7 * 9 + 6\n9 * 3 * ((3 * 6 + 4 + 8) + 9 + 2) * 3\n8 * 3 + 6 * 8 * 2 + 4"
  # "1 + 2 * 3 + 4 * 5 + 6\n1 + (2 * 3) + (4 * (5 + 6))\n2 * 3 + (4 * 5)\n5 + (8 * 3 + 9 + 3 * 4 * 3)\n5 * 9 * (7 * 3 * 3 + 9 * 3 + (8 + 6 * 4))\n((2 + 4 * 9) * (6 + 9 * 8 + 6) + 6) + 2 + 4 * 2"
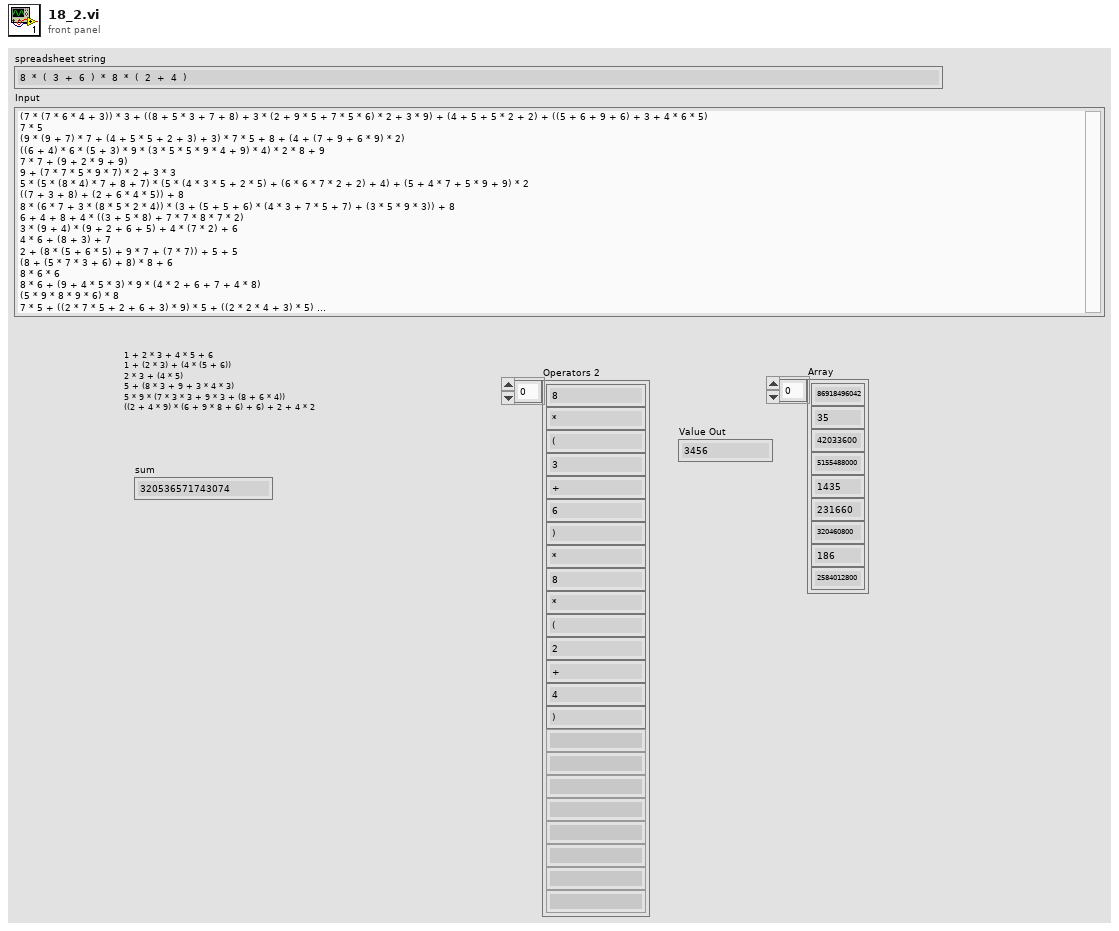
[diagram p1: front panel]
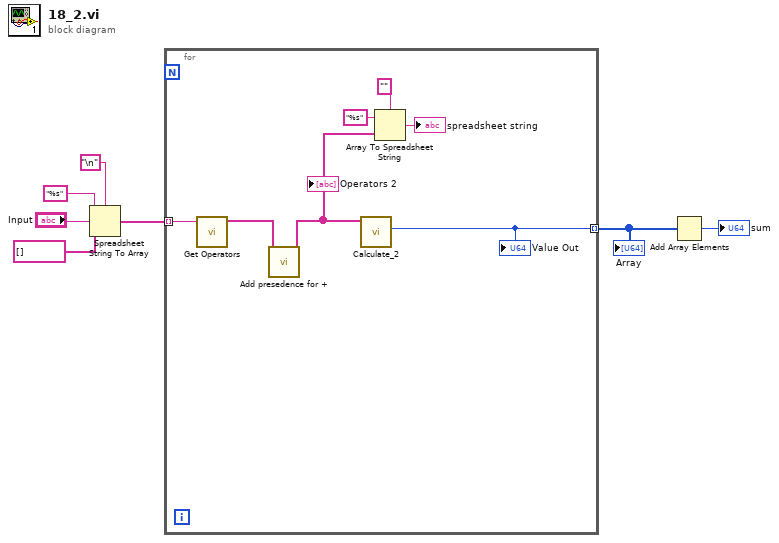
[diagram p0: block diagram]
diagram:
  n1 = Spreadsheet String To Array(delimiter (Tab)="\n", format string="%s", spreadsheet string="Input", array type (2D Dbl)=string[] []) -> (array=w3:string[])
  n2 = for {
    tunnel: w3 -> [w14] mode=indexing
    tunnel: [w13] -> w2 mode=indexing
    n3 = call "Get Operators.vi"("Expression"=w14) -> ("Operators"=w12:string[])  [unwired: 10 in]
    n4 = call "Add presedence for +.vi"("Operators"=w12) -> ("Operators 2"=w11:string[])  [unwired: 10 in]
    "Operators 2" <- w11
    n5 = call "Calculate_2.vi"("Operators"=w11) -> ("Value Out"=w13:u64)  [unwired: 9 in, 1 out]
    "Value Out" <- w13
    n6 = Array To Spreadsheet String(delimiter (Tab)="", array=w11, 3:"%s") -> (spreadsheet string=→"spreadsheet string":string)
  }
  "Array" <- w2
  n7 = Add Array Elements(numeric array=w2) -> (sum=→"sum":u64)
